vi "41 rec.vi"() -> ()   [LabVIEW 2014]
uses:
  <vilib>/LabVIEW Targets/FPGA/cRIO/shared/nicrio_ModuleControls/nicrio_cRIO-9467_Altitude.ctl
  <vilib>/LabVIEW Targets/FPGA/cRIO/shared/nicrio_ModuleControls/nicrio_cRIO-9467_Longitude.ctl
  <vilib>/LabVIEW Targets/FPGA/cRIO/shared/nicrio_ModuleControls/nicrio_cRIO-9467_Latitude.ctl
  <vilib>/LabVIEW Targets/FPGA/cRIO/shared/nicrio_ModuleControls/nicrio_cRIO-9225_DataRatesRing.ctl
  <vilib>/LabVIEW Targets/FPGA/cRIO/shared/nicrio_ModuleControls/nicrio_cRIO-9227_DataRatesRing.ctl
  <vilib>/rvi/FXPMathLib/FxpSinAndCos/subVIs/nifxpmath_SinAndCos_SimConfig.ctl
  <vilib>/rvi/FXPMathLib/FxpRectToPolar/subVIs/nifxpmath_RectToPolar_SimConfig.ctl
  <vilib>/rvi/Emulation/niFpgaGetClockAttributes.vi
  <vilib>/rvi/Emulation/niFpgaSctlEmulationGetInTimedLoop.vi
  <vilib>/rvi/Emulation/niFpgaEmulationReportErrorSimple.vi
  <vilib>/rvi/eio/common/nirviEmuTemplateMethod_errors.vi
  <vilib>/rvi/eio/common/nirviEmuTemplatePropertyGet_noerrors.vi
  <vilib>/rvi/Emulation/niFpgaCriticalErrorInLSC.vi
  <vilib>/rvi/Memory/Memory_Emulation/nirvimemoryFastEmulation.vi
  <vilib>/rvi/Memory/Memory_Emulation/nirvimemoryEmulation.vi
  <vilib>/rvi/Emulation/niFpgaEmulationIsFPGAContextNoSignature.vi
  <vilib>/rvi/DataTransferAndStorage/Container/Common/niFpgaContainerGetUniqueNameForEmu.vi
  <vilib>/rvi/Emulation/niFpgaProcessEmulError.vi
  <vilib>/rvi/errors/nirviReportUnexpectedCaseInternalError (U32).vi
  <vilib>/rvi/FXPMathLib/FxpSinAndCos/simVIs/DllFxpSinAndCosTemp_sub.vi
  <vilib>/rvi/FXPMathLib/FxpRectToPolar/simVIs/DllFxpRectToPolarTemp_sub.vi
  <vilib>/rvi/eio/common/nirviEmuTemplatePropertyGet_errors.vi
  <vilib>/rvi/DataTransferAndStorage/Container/Common/niFpgaContainerSetEmuInfo.vi
  <vilib>/rvi/eio/common/nirviEmuReportErrorAndStop.vi
  <vilib>/rvi/eio/common/nirviEmuTemplatePropertySet_noerrors.vi
  <vilib>/eio/EIOMethodNode/EIOMethodNode.xnode
  <vilib>/eio/EIOPropertyNode/EIOPropertyNode.xnode
  <vilib>/eio/EIONode/EIONode.xnode
  <vilib>/rvi/DataTransferAndStorage/Container/XNode/niFpgaContainer.xnode
  <vilib>/rvi/FXPMathLib/FxpMul/XNode/nifxpmath_Multiplier.xnode
  <vilib>/rvi/FXPMathLib/FxpSinAndCos/XNode/nifxpmath_SinAndCos.xnode
  <vilib>/rvi/FXPMathLib/FxpAdd/XNode/nifxpmath_Add.xnode
  <vilib>/rvi/FXPMathLib/FxpSub/XNode/nifxpmath_Sub.xnode
  <vilib>/rvi/FXPMathLib/FxpRectToPolar/XNode/nifxpmath_RectToPolar.xnode
  <vilib>/rvi/LocalResourceManager/LocalResourceManager.xnode
  <vilib>/rvi/FXPMathLib/sim/FxpSim.dll
  akhil/fpga timekeeper/FPGA Timekeeper.lvlib
  <vilib>/rvi/eio/common/nirviEmuTemplatePropertySet_errors.vi
panel:
  out "angles":fxp<+/-,22,10>[](array[numeric])
  out "Array":T1(array[cluster])
  out "magnitude":fxp<+,60,17>[](array[numeric])
  out "Firmware Version":u32 format="%.0x"
  out "Vendor ID":u16 format="%.0x"
  out "Module ID":u16 format="%.0x"
  out "Serial Number":u32 format="%.0x"
  out "FPGA Error Out":errorcluster
  in  "stop 2":bool
  out "PPS Timestamp (TAI)":u64
  out "UTC Offset":i8
  out "UTC Offset Valid":bool
  out "GPS Status":T2(ring)
  out "Antenna Status":T3(ring)
  out "Leap Second Direction":enum8{"Add", "Delete"}(ring)
  out "Leap Second Pending":bool
  out "Leap Second Occurred":bool
  out "Satellites Available":u8
  out "Self-Survey Complete":bool
  out "Latitude (°)":T4 format="%.6f"
  out "Longitude (°)":T5 format="%.6g"
  out "Altitude (m)":T6 format="%.2f"
  out "Timed Out":bool
  out "Iterations":i32
  out "FPGA Timekeeper time (ns) 2":u64
  out "GPS status":T2(ring)
  out "FPGA Timekeeper locked":bool
  out "offset from time reference":i32
  out "antenna status":T3(ring)
  out "satellites available":u8
  out "UTC offset":i8
  out "UTC offset valid":bool
  out "ROCOF voltage":fxp<+/-,26,12>
  out "ROCOF current":fxp<+/-,26,12>
  out "DIFFERENCE IN ANGLES":fxp<+/-,26,12>
  out "DIFFERENCE IN ANGLES 2":fxp<+/-,26,12>
  out "Voltage Frequency":fxp<+/-,49,18>
  out "Current Frequency":fxp<+/-,49,18>
  in  "stop":bool
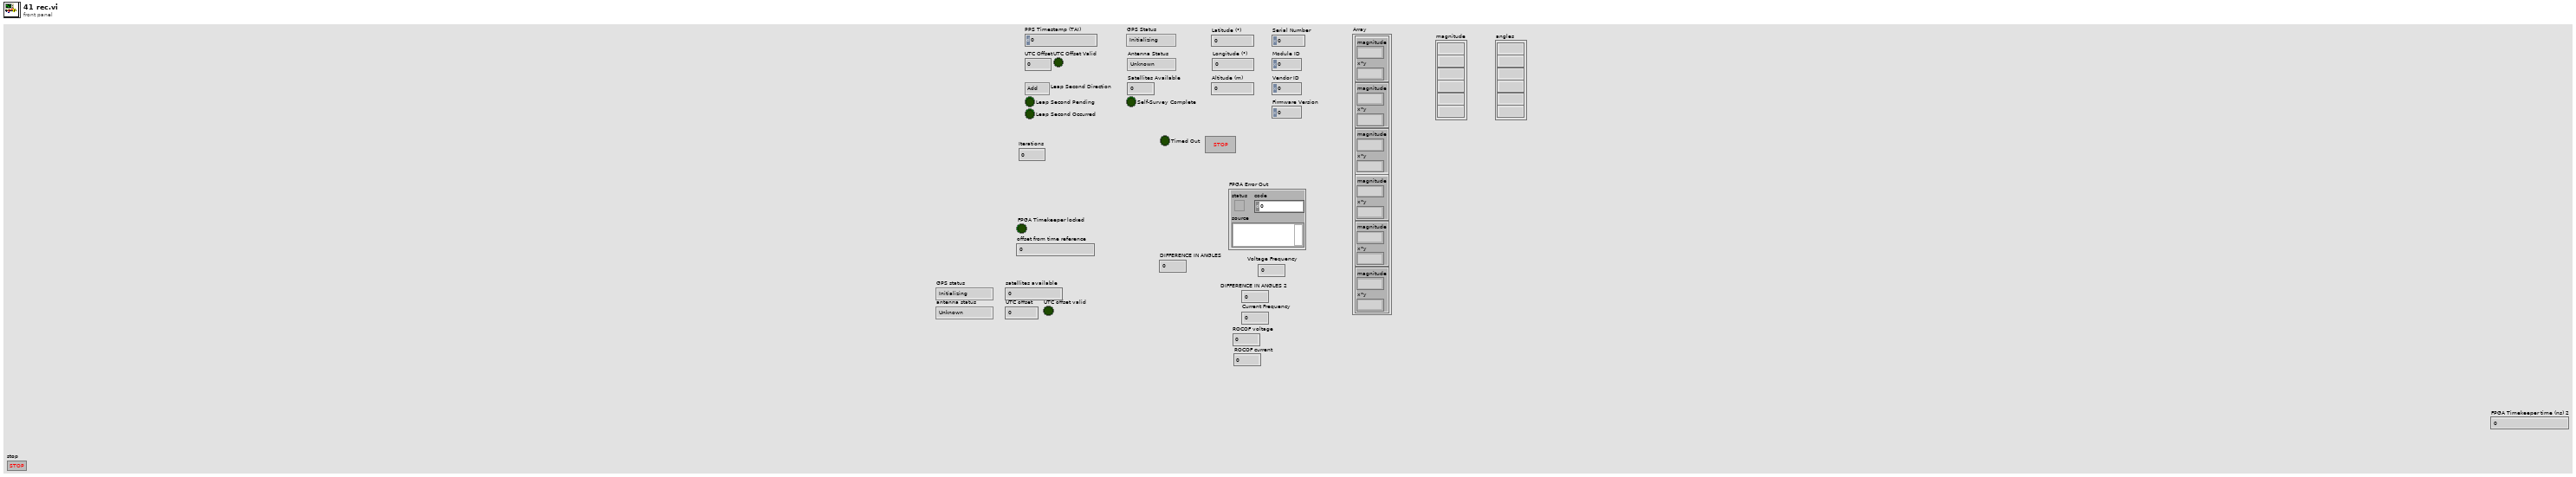
[diagram p1: front panel]
types:
  T1 = cluster{"magnitude":fxp<+,60,17>, "x*y":fxp<+/-,22,10>}[]
  T2 = enum8{"Initializing", "Normal", "Unable to get fix"}
  T3 = enum8{"Unknown", "Normal", "Absent", "Overcurrent"}
  T4 = typedef "nicrio_cRIO-9467_Latitude.ctl" = fxp<+/-,28,8>
  T5 = typedef "nicrio_cRIO-9467_Longitude.ctl" = fxp<+/-,29,9>
  T6 = typedef "nicrio_cRIO-9467_Altitude.ctl" = fxp<+/-,24,17>
  T7 = typedef "nicrio_cRIO-9227_DataRatesRing.ctl" = u8
  T8 = typedef "nicrio_cRIO-9225_DataRatesRing.ctl" = u8
  T9 = cluster{"magnitude":fxp<+,60,17>, "x*y":fxp<+/-,22,10>}
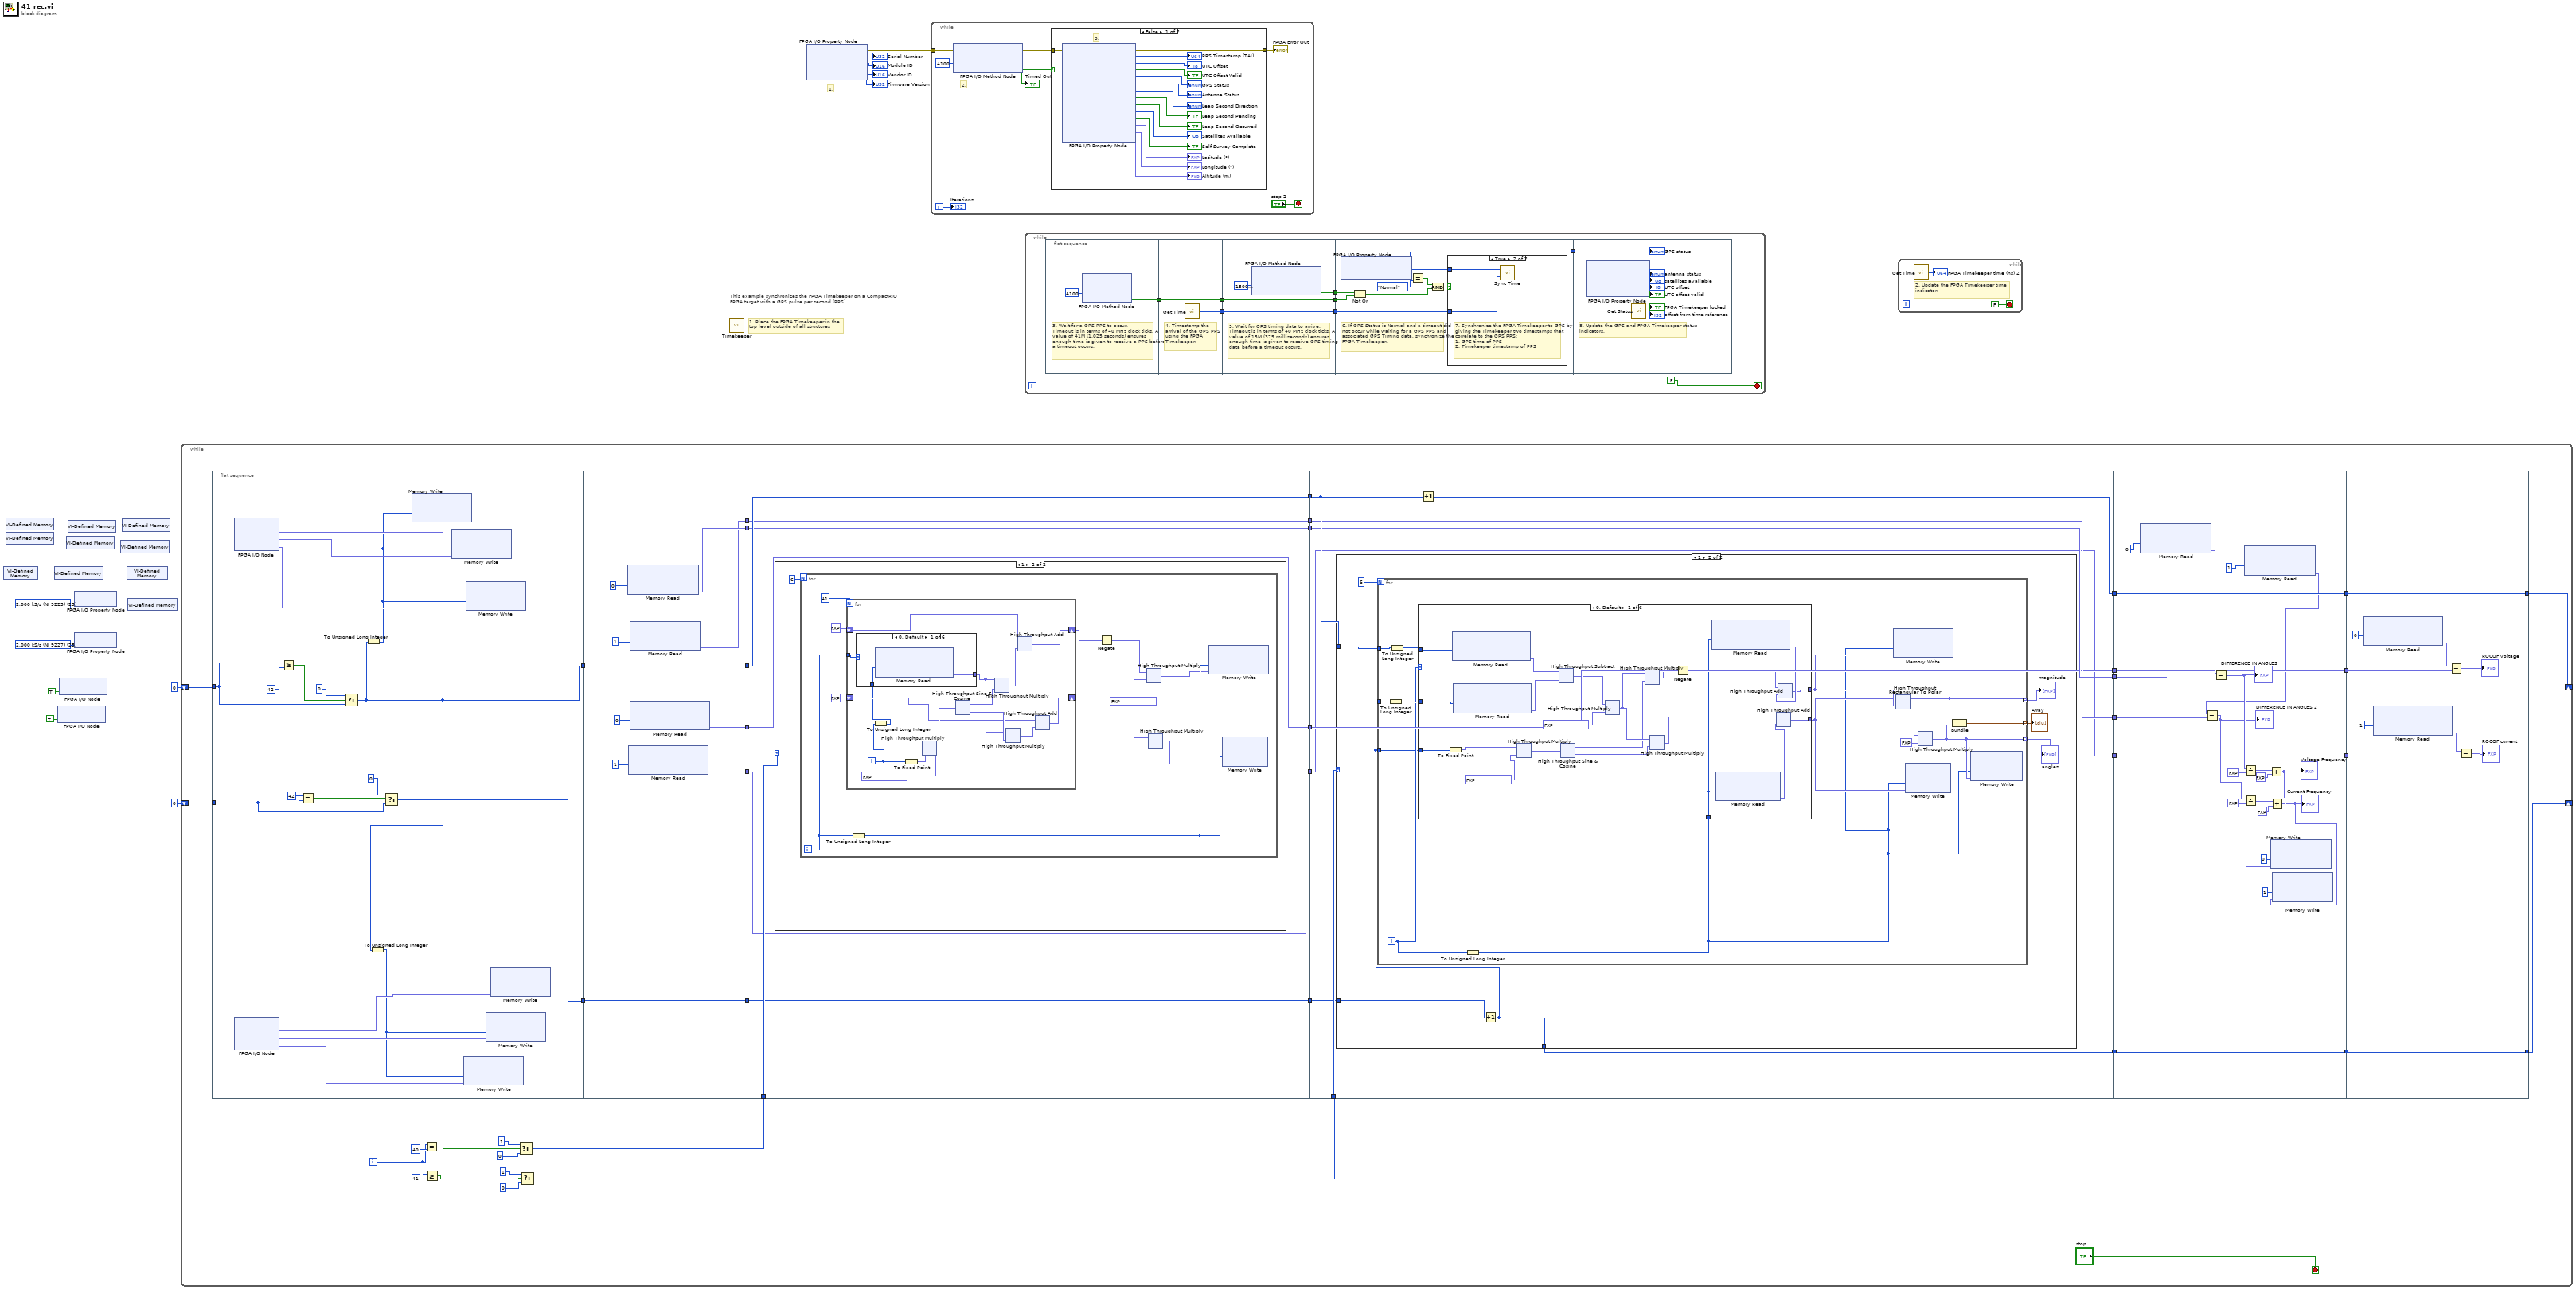
[diagram p0: block diagram]
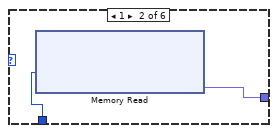
[diagram p5: hidden frame]
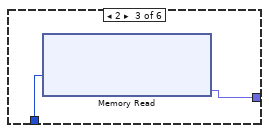
[diagram p6: hidden frame]
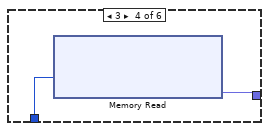
[diagram p7: hidden frame]
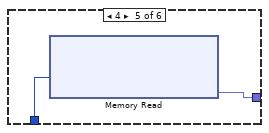
[diagram p8: hidden frame]
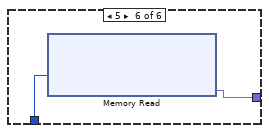
[diagram p9: hidden frame]
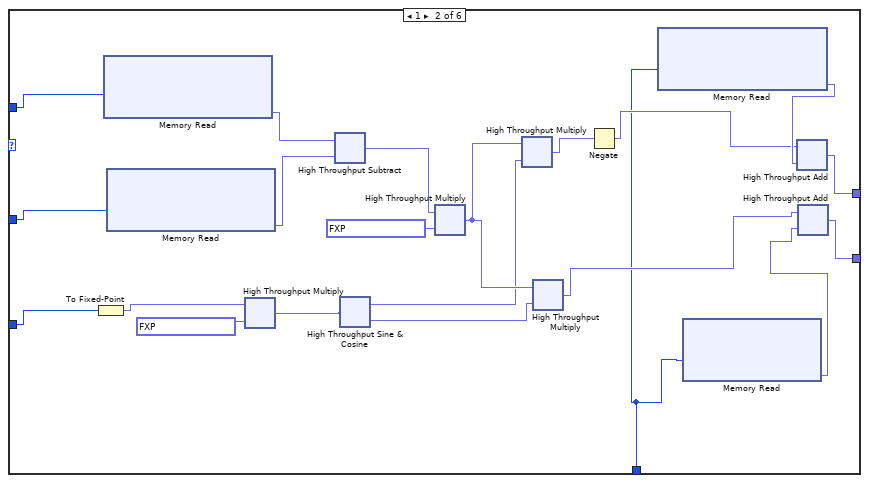
[diagram p11: hidden frame]
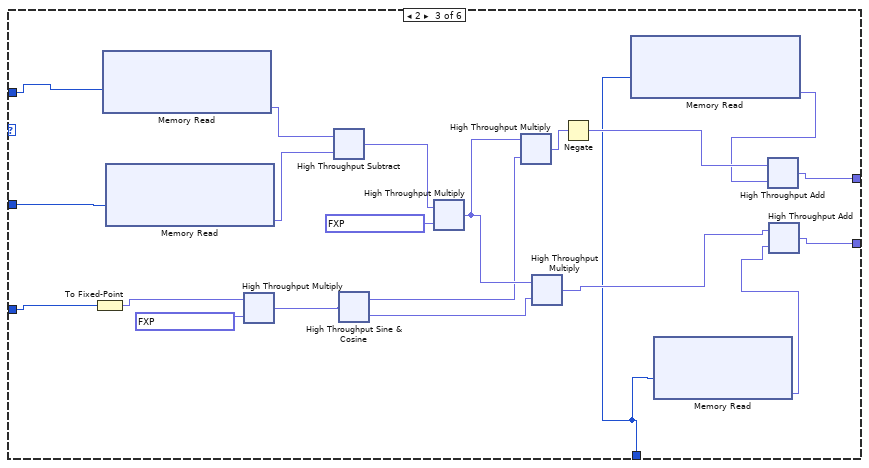
[diagram p12: hidden frame]
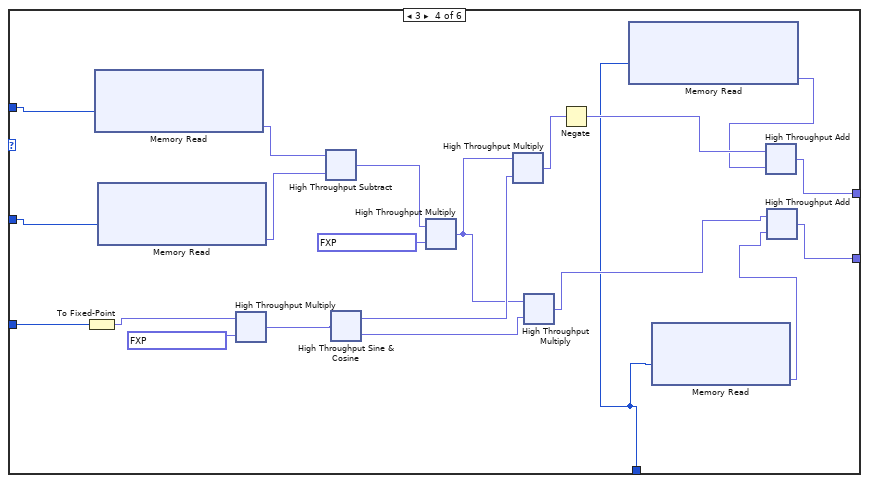
[diagram p13: hidden frame]
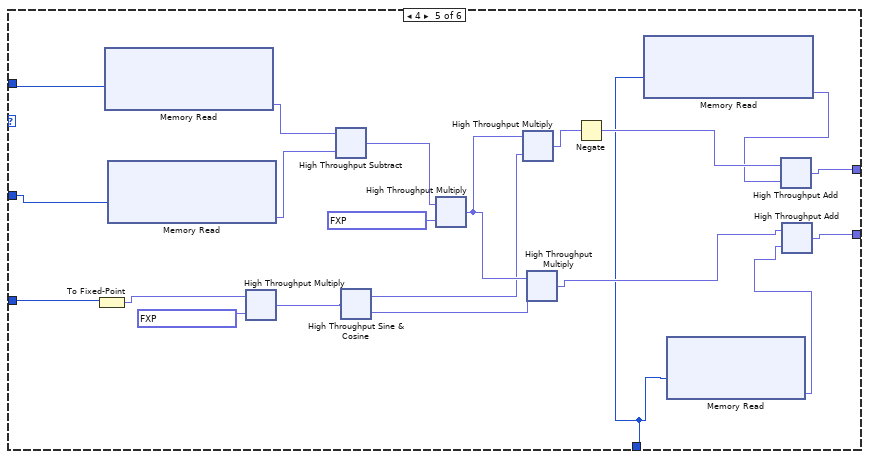
[diagram p14: hidden frame]
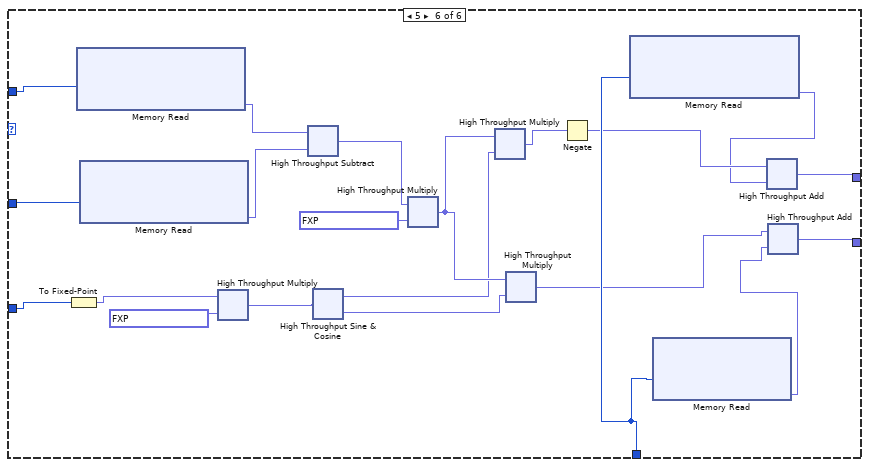
[diagram p15: hidden frame]
diagram:
  w5 = T7 25 items=["50.000 kS/s (NI 9227)"=1, "25.000 kS/s (NI 9227)"=2, "16.667 kS/s (NI 9227)"=3, "12.500 kS/s (NI 9227)"=4, "10.000 kS/s (NI 9227)"=5, "8.333 kS/s (NI 9227)"=6, "7.143 kS/s (NI 9227)"=7, "6.250 kS/s (NI 9227)"=8, "5.556 kS/s (NI 9227)"=9, "5.000 kS/s (NI 9227)"=10, "4.545 kS/s (NI 9227)"=11, "4.167 kS/s (NI 9227)"=12, "3.846 kS/s (NI 9227)"=13, "3.571 kS/s (NI 9227)"=14, "3.333 kS/s (NI 9227)"=15, "3.125 kS/s (NI 9227)"=16, "2.941 kS/s (NI 9227)"=17, "2.778 kS/s (NI 9227)"=18, "2.632 kS/s (NI 9227)"=19, "2.500 kS/s (NI 9227)"=20, "2.381 kS/s (NI 9227)"=21, "2.273 kS/s (NI 9227)"=22, "2.174 kS/s (NI 9227)"=23, "2.083 kS/s (NI 9227)"=24, "2.000 kS/s (NI 9227)"=25, "1.923 kS/s (NI 9227)"=26, "1.852 kS/s (NI 9227)"=27, "1.786 kS/s (NI 9227)"=28, "1.724 kS/s (NI 9227)"=29, "1.667 kS/s (NI 9227)"=30, "1.613 kS/s (NI 9227)"=31] ("Data Rate")
  w6 = T8 25 items=["50.000 kS/s (NI 9225)"=1, "25.000 kS/s (NI 9225)"=2, "16.667 kS/s (NI 9225)"=3, "12.500 kS/s (NI 9225)"=4, "10.000 kS/s (NI 9225)"=5, "8.333 kS/s (NI 9225)"=6, "7.143 kS/s (NI 9225)"=7, "6.250 kS/s (NI 9225)"=8, "5.556 kS/s (NI 9225)"=9, "5.000 kS/s (NI 9225)"=10, "4.545 kS/s (NI 9225)"=11, "4.167 kS/s (NI 9225)"=12, "3.846 kS/s (NI 9225)"=13, "3.571 kS/s (NI 9225)"=14, "3.333 kS/s (NI 9225)"=15, "3.125 kS/s (NI 9225)"=16, "2.941 kS/s (NI 9225)"=17, "2.778 kS/s (NI 9225)"=18, "2.632 kS/s (NI 9225)"=19, "2.500 kS/s (NI 9225)"=20, "2.381 kS/s (NI 9225)"=21, "2.273 kS/s (NI 9225)"=22, "2.174 kS/s (NI 9225)"=23, "2.083 kS/s (NI 9225)"=24, "2.000 kS/s (NI 9225)"=25, "1.923 kS/s (NI 9225)"=26, "1.852 kS/s (NI 9225)"=27, "1.786 kS/s (NI 9225)"=28, "1.724 kS/s (NI 9225)"=29, "1.667 kS/s (NI 9225)"=30, "1.613 kS/s (NI 9225)"=31] ("Data Rate")
  # "1."
  # "This example synchronizes the FPGA Timekeeper on a CompactRIO FPGA target with a GPS pulse per second (PPS)."
  # "1. Place the FPGA Timekeeper in the\ntop level outside of all structures"
  n1 = xnode "VI-Defined Memory"() -> ()  [unwired: 1 out]
  n2 = xnode "VI-Defined Memory"() -> ()  [unwired: 1 out]
  n3 = xnode "VI-Defined Memory"() -> ()  [unwired: 1 out]
  n4 = xnode "VI-Defined Memory"() -> ()  [unwired: 1 out]
  n5 = xnode "FPGA I/O Node"("Mod2/Start"=TRUE) -> ()  [unwired: 1 in, 1 out]
  n6 = xnode "FPGA I/O Node"("Mod1/Start"=TRUE) -> ()  [unwired: 1 in, 1 out]
  n7 = xnode "VI-Defined Memory"() -> ()  [unwired: 1 out]
  n8 = xnode "VI-Defined Memory"() -> ()  [unwired: 1 out]
  n9 = xnode "FPGA I/O Property Node"("Data Rate"=w6) -> ()  [unwired: 1 in, 1 out]
  n10 = xnode "FPGA I/O Property Node"("Data Rate"=w5) -> ()  [unwired: 1 in, 1 out]
  n11 = xnode "VI-Defined Memory"() -> ()  [unwired: 1 out]
  n12 = xnode "VI-Defined Memory"() -> ()  [unwired: 1 out]
  n13 = xnode "VI-Defined Memory"() -> ()  [unwired: 1 out]
  n14 = xnode "VI-Defined Memory"() -> ()  [unwired: 1 out]
  n15 = while {
    shift-right: [w50] -> _
    shift-left: 0 -> [w51]
    shift-right: [w34] -> _
    shift-left: 0 ("t") -> [w36]
    i -> [w41]
    stop <- "stop" stop-if-true
    n16 = flat-sequence {
      tunnel: w51 -> [w58]
      tunnel: [w52] -> w31
      tunnel: w36 -> [w54]
      tunnel: [w53] -> w29
      tunnel: w31 -> [w79]
      tunnel: [w79] -> w30
      tunnel: w29 -> [w78]
      tunnel: [w78] -> w28
      tunnel: [w75] -> w25
      tunnel: [w74] -> w22
      tunnel: [w71] -> w16
      tunnel: [w70] -> w12
      tunnel: w30 -> [w86]
      tunnel: w40 -> [w85]
      tunnel: [w86] -> w39
      tunnel: [w84] -> w35
      tunnel: w28 -> [w84]
      tunnel: [w83] -> w26
      tunnel: w25 -> [w83]
      tunnel: [w82] -> w23
      tunnel: w22 -> [w82]
      tunnel: [w81] -> w17
      tunnel: w16 -> [w81]
      tunnel: [w80] -> w13
      tunnel: w12 -> [w80]
      tunnel: w39 -> [w162]
      tunnel: w38 -> [w164]
      tunnel: w35 -> [w161]
      tunnel: [w163] -> w33
      tunnel: [w160] -> w32
      tunnel: [w159] -> w27
      tunnel: w26 -> [w159]
      tunnel: [w158] -> w24
      tunnel: w23 -> [w158]
      tunnel: [w157] -> w18
      tunnel: w17 -> [w157]
      tunnel: [w156] -> w14
      tunnel: w13 -> [w156]
      tunnel: w33 -> [w551]
      tunnel: w32 -> [w550]
      tunnel: w27 -> [w540]
      tunnel: w24 -> [w530]
      tunnel: [w551] -> w21
      tunnel: [w550] -> w20
      tunnel: [w533] -> w19
      tunnel: w18 -> [w533]
      tunnel: [w532] -> w15
      tunnel: w14 -> [w532]
      tunnel: [w560] -> w34
      tunnel: [w561] -> w50
      tunnel: w21 -> [w561]
      tunnel: w20 -> [w560]
      tunnel: w19 -> [w555]
      tunnel: w15 -> [w554]
      frame #0 {
        n17 = xnode "FPGA I/O Node"() -> ("Mod1/AI0"=w66:fxp<+/-,24,10>, "Mod1/AI1"=w62:fxp<+/-,24,10>, "Mod1/AI2"=w65:fxp<+/-,24,10>)  [unwired: 3 in, 3 out]
        n18 = xnode "FPGA I/O Node"() -> ("Mod2/AI0"=w69:fxp<+/-,24,5>, "Mod2/AI1"=w68:fxp<+/-,24,5>, "Mod2/AI2"=w67:fxp<+/-,24,5>)  [unwired: 3 in, 3 out]
        n19 = Greater Or Equal?(x=w58, y=42 ("x")) -> (x >= y?=w64:bool)
        n20 = Equal?(x=42, y=w54) -> (x = y?=w56:bool)
        n21 = Select(t=0, s=w64, f=w58) -> (s? t:f=w52:i32)
        n22 = To Unsigned Long Integer(number=w52) -> (unsigned 32bit integer=w61:u32)
        n23 = To Unsigned Long Integer(number=w52) -> (unsigned 32bit integer=w60:u32)
        n24 = Select(t=0, s=w56, f=w54) -> (s? t:f=w53:i32)
        n25 = xnode ("Memory Write")("Address"=w61, "Data"=w66) -> ()  [unwired: 1 in, 1 out]
        n26 = xnode ("Memory Write")("Address"=w61, "Data"=w62) -> ()  [unwired: 1 in, 1 out]
        n27 = xnode ("Memory Write")("Address"=w60, "Data"=w67) -> ()  [unwired: 1 in, 1 out]
        n28 = xnode ("Memory Write")("Address"=w61, "Data"=w65) -> ()  [unwired: 1 in, 1 out]
        n29 = xnode ("Memory Write")("Address"=w60, "Data"=w68) -> ()  [unwired: 1 in, 1 out]
        n30 = xnode ("Memory Write")("Address"=w60, "Data"=w69) -> ()  [unwired: 1 in, 1 out]
      }
      frame #1 {
        n31 = xnode ("Memory Read")("Address"=u32 0) -> ("Data"=w75:fxp<+/-,25,11>)  [unwired: 1 in, 1 out]
        n32 = xnode ("Memory Read")("Address"=u32 1) -> ("Data"=w70:fxp<+/-,25,11>)  [unwired: 1 in, 1 out]
        n33 = xnode ("Memory Read")("Address"=u32 1) -> ("Data"=w74:fxp<+/-,25,11>)  [unwired: 1 in, 1 out]
        n34 = xnode ("Memory Read")("Address"=u32 0) -> ("Data"=w71:fxp<+/-,25,11>)  [unwired: 1 in, 1 out]
      }
      frame #2 {
        n35 = case shown="1" w85 {
          frame 0, Default {
          }
          frame 1 {
            n36 = for {
              N: 6 -> [_]
              i -> [w94]
              w88 = fxp<+/-,16,1> 0.03533935546875 ("y")
              n37 = for {
                N: 41 -> [_]
                shift-right: [w106] -> w92
                shift-left: fxp<+/-,44,16> 0.0 ("x+y") -> [w105]
                shift-right: [w109] -> w95
                shift-left: fxp<+/-,42,14> 0.0 ("x+y") -> [w104]
                tunnel: w94 -> [w103]
                i -> [w101]
                n38 = To Unsigned Long Integer(number=w101) -> (unsigned 32bit integer=w100:u32)
                n39 = case shown="0, Default" w103 {
                  tunnel: [w115 w116 w118 w120 w122 w125] -> w102
                  tunnel: w100 -> [w114 w117 w119 w121 w123 w124]
                  frame 0, Default {
                    n40 = xnode ("Memory Read")("Address"=w114) -> ("Data"=w115:fxp<+/-,25,11>)  [unwired: 1 in, 1 out]
                  }
                  frame 1 {
                    n41 = xnode ("Memory Read")("Address"=w117) -> ("Data"=w116:fxp<+/-,25,11>)  [unwired: 1 in, 1 out]
                  }
                  frame 2 {
                    n42 = xnode ("Memory Read")("Address"=w119) -> ("Data"=w118:fxp<+/-,25,11>)  [unwired: 1 in, 1 out]
                  }
                  frame 3 {
                    n43 = xnode ("Memory Read")("Address"=w121) -> ("Data"=w120:fxp<+/-,25,11>)  [unwired: 1 in, 1 out]
                  }
                  frame 4 {
                    n44 = xnode ("Memory Read")("Address"=w123) -> ("Data"=w122:fxp<+/-,25,11>)  [unwired: 1 in, 1 out]
                  }
                  frame 5 {
                    n45 = xnode ("Memory Read")("Address"=w124) -> ("Data"=w125:fxp<+/-,25,11>)  [unwired: 1 in, 1 out]
                  }
                }
                n46 = To Fixed-Point(number=w101) -> (fixed-point=w113:fxp<+/-,32,32>)  [unwired: 1 in]
                n47 = xnode ("High Throughput Multiply")("x"=fxp<+/-,32,16> 0.04998779296875 ("number"), "y"=w113) -> ("x*y"=w112:fxp<+/-,64,48>)
                n48 = xnode "High Throughput Sine & Cosine"("x (pi)"=w112) -> ("sin(x)"=w111:fxp<+/-,16,2>, "cos(x)"=w108:fxp<+/-,16,2>)
                n49 = xnode ("High Throughput Multiply")("x"=w102, "y"=w111) -> ("x*y"=w110:fxp<+/-,41,13>)
                n50 = xnode ("High Throughput Multiply")("x"=w102, "y"=w108) -> ("x*y"=w107:fxp<+/-,41,13>)
                n51 = xnode ("High Throughput Add")("x"=w104, "y"=w110) -> ("x+y"=w109:fxp<+/-,42,14>)
                n52 = xnode ("High Throughput Add")("x"=w105, "y"=w107) -> ("x+y"=w106:fxp<+/-,44,16>)
              }
              n53 = To Unsigned Long Integer(number=w94) -> (unsigned 32bit integer=w93:u32)
              n54 = Negate(x=w95) -> (-x=w91:fxp<+/-,43,15>)
              n55 = xnode ("High Throughput Multiply")("x"=w91, "y"=w88) -> ("x*y"=w89:fxp<+/-,59,16>)
              n56 = xnode ("High Throughput Multiply")("x"=w88, "y"=w92) -> ("x*y"=w90:fxp<+/-,60,17>)
              n57 = xnode ("Memory Write")("Address"=w93, "Data"=w89) -> ()  [unwired: 1 in, 1 out]
              n58 = xnode ("Memory Write")("Address"=w93, "Data"=w90) -> ()  [unwired: 1 in, 1 out]
            }
          }
        }
      }
      frame #3 {
        n59 = case shown="1" w164 {
          tunnel: w162 -> [_ w171]
          tunnel: w161 -> [w165 w167]
          tunnel: [w165 w166] -> w160
          frame 0, Default {
          }
          frame 1 {
            n60 = Increment(x=w167) -> (x+1=w166:i32)
            n61 = for {
              N: 6 -> [_]
              tunnel: w171 -> [w186]
              tunnel: [w178] -> w170 mode=indexing
              tunnel: [w174] -> w168 mode=indexing
              tunnel: [w177] -> w169 mode=indexing
              tunnel: w166 -> [w176]
              tunnel: w166 -> [w175]
              i -> [w183]
              n62 = To Unsigned Long Integer(number=w176) -> (unsigned 32bit integer=w184:u32)
              n63 = To Unsigned Long Integer(number=w186) -> (unsigned 32bit integer=w185:u32)
              n64 = To Unsigned Long Integer(number=w183) -> (unsigned 32bit integer=w173:u32)
              n65 = case shown="0, Default" w183 {
                tunnel: w185 -> [w244 w284 w335 w386 w438 w488]
                tunnel: w184 -> [w243 w283 w336 w387 w437 w487]
                tunnel: w173 -> [w230 w278 w329 w380 w431 w486]
                tunnel: [w228 w277 w328 w379 w430 w481] -> w180
                tunnel: [w227 w276 w327 w378 w429 w480] -> w179
                tunnel: w175 -> [w226 w275 w326 w377 w428 w479]
                frame 0, Default {
                  n66 = To Fixed-Point(number=w226) -> (fixed-point=w237:fxp<+/-,32,32>)  [unwired: 1 in]
                  n67 = xnode ("Memory Read")("Address"=w244) -> ("Data"=w235:fxp<+/-,25,11>)  [unwired: 1 in, 1 out]
                  n68 = xnode ("Memory Read")("Address"=w243) -> ("Data"=w234:fxp<+/-,25,11>)  [unwired: 1 in, 1 out]
                  n69 = xnode ("High Throughput Multiply")("x"=w237, "y"=fxp<+/-,32,16> 0.04998779296875 ("number")) -> ("x*y"=w236:fxp<+/-,64,48>)
                  n70 = xnode "High Throughput Subtract"("x"=w235, "y"=w234) -> ("x-y"=w242:fxp<+/-,26,12>)
                  n71 = xnode "High Throughput Sine & Cosine"("x (pi)"=w236) -> ("sin(x)"=w239:fxp<+/-,16,2>, "cos(x)"=w238:fxp<+/-,16,2>)
                  n72 = xnode ("High Throughput Multiply")("x"=w242, "y"=fxp<+/-,16,1> 0.03533935546875) -> ("x*y"=w241:fxp<+/-,42,13>)
                  n73 = xnode ("High Throughput Multiply")("x"=w241, "y"=w239) -> ("x*y"=w240:fxp<+/-,58,15>)
                  n74 = xnode ("High Throughput Multiply")("x"=w241, "y"=w238) -> ("x*y"=w229:fxp<+/-,58,15>)
                  n75 = Negate(x=w240) -> (-x=w231:fxp<+/-,59,16>)
                  n76 = xnode ("Memory Read")("Address"=w230) -> ("Data"=w232:fxp<+/-,25,11>)  [unwired: 1 in, 1 out]
                  n77 = xnode ("Memory Read")("Address"=w230) -> ("Data"=w233:fxp<+/-,25,11>)  [unwired: 1 in, 1 out]
                  n78 = xnode ("High Throughput Add")("x"=w229, "y"=w233) -> ("x+y"=w227:fxp<+/-,59,16>)
                  n79 = xnode ("High Throughput Add")("x"=w231, "y"=w232) -> ("x+y"=w228:fxp<+/-,60,17>)
                }
                frame 1 {
                  n80 = To Fixed-Point(number=w275) -> (fixed-point=w289:fxp<+/-,32,32>)  [unwired: 1 in]
                  n81 = xnode ("Memory Read")("Address"=w284) -> ("Data"=w286:fxp<+/-,25,11>)  [unwired: 1 in, 1 out]
                  n82 = xnode ("Memory Read")("Address"=w283) -> ("Data"=w285:fxp<+/-,25,11>)  [unwired: 1 in, 1 out]
                  n83 = xnode ("High Throughput Multiply")("x"=w289, "y"=fxp<+/-,16,1> 0.04998779296875) -> ("x*y"=w287:fxp<+/-,48,33>)
                  n84 = xnode "High Throughput Subtract"("x"=w286, "y"=w285) -> ("x-y"=w295:fxp<+/-,26,12>)
                  n85 = xnode "High Throughput Sine & Cosine"("x (pi)"=w287) -> ("sin(x)"=w291:fxp<+/-,16,2>, "cos(x)"=w290:fxp<+/-,16,2>)
                  n86 = xnode ("High Throughput Multiply")("x"=w295, "y"=fxp<+/-,16,1> 0.03533935546875) -> ("x*y"=w293:fxp<+/-,42,13>)
                  n87 = xnode ("High Throughput Multiply")("x"=w293, "y"=w291) -> ("x*y"=w292:fxp<+/-,58,15>)
                  n88 = xnode ("High Throughput Multiply")("x"=w293, "y"=w290) -> ("x*y"=w279:fxp<+/-,58,15>)
                  n89 = Negate(x=w292) -> (-x=w280:fxp<+/-,59,16>)
                  n90 = xnode ("Memory Read")("Address"=w278) -> ("Data"=w281:fxp<+/-,25,11>)  [unwired: 1 in, 1 out]
                  n91 = xnode ("Memory Read")("Address"=w278) -> ("Data"=w282:fxp<+/-,25,11>)  [unwired: 1 in, 1 out]
                  n92 = xnode ("High Throughput Add")("x"=w280, "y"=w281) -> ("x+y"=w277:fxp<+/-,60,17>)
                  n93 = xnode ("High Throughput Add")("x"=w279, "y"=w282) -> ("x+y"=w276:fxp<+/-,59,16>)
                }
                frame 2 {
                  n94 = To Fixed-Point(number=w326) -> (fixed-point=w341:fxp<+/-,32,32>)  [unwired: 1 in]
                  n95 = xnode ("Memory Read")("Address"=w335) -> ("Data"=w338:fxp<+/-,25,11>)  [unwired: 1 in, 1 out]
                  n96 = xnode ("Memory Read")("Address"=w336) -> ("Data"=w337:fxp<+/-,25,11>)  [unwired: 1 in, 1 out]
                  n97 = xnode ("High Throughput Multiply")("x"=w341, "y"=fxp<+/-,16,1> 0.04998779296875) -> ("x*y"=w339:fxp<+/-,48,33>)
                  n98 = xnode "High Throughput Subtract"("x"=w338, "y"=w337) -> ("x-y"=w346:fxp<+/-,26,12>)
                  n99 = xnode "High Throughput Sine & Cosine"("x (pi)"=w339) -> ("sin(x)"=w343:fxp<+/-,16,2>, "cos(x)"=w342:fxp<+/-,16,2>)
                  n100 = xnode ("High Throughput Multiply")("x"=w346, "y"=fxp<+/-,16,1> 0.03533935546875) -> ("x*y"=w344:fxp<+/-,42,13>)
                  n101 = xnode ("High Throughput Multiply")("x"=w344, "y"=w343) -> ("x*y"=w331:fxp<+/-,58,15>)
                  n102 = xnode ("High Throughput Multiply")("x"=w344, "y"=w342) -> ("x*y"=w330:fxp<+/-,58,15>)
                  n103 = Negate(x=w331) -> (-x=w334:fxp<+/-,59,16>)
                  n104 = xnode ("Memory Read")("Address"=w329) -> ("Data"=w332:fxp<+/-,25,11>)  [unwired: 1 in, 1 out]
                  n105 = xnode ("Memory Read")("Address"=w329) -> ("Data"=w333:fxp<+/-,25,11>)  [unwired: 1 in, 1 out]
                  n106 = xnode ("High Throughput Add")("x"=w334, "y"=w332) -> ("x+y"=w328:fxp<+/-,60,17>)
                  n107 = xnode ("High Throughput Add")("x"=w330, "y"=w333) -> ("x+y"=w327:fxp<+/-,59,16>)
                }
                frame 3 {
                  n108 = To Fixed-Point(number=w377) -> (fixed-point=w393:fxp<+/-,32,32>)  [unwired: 1 in]
                  n109 = xnode ("Memory Read")("Address"=w386) -> ("Data"=w396:fxp<+/-,25,11>)  [unwired: 1 in, 1 out]
                  n110 = xnode ("Memory Read")("Address"=w387) -> ("Data"=w397:fxp<+/-,25,11>)  [unwired: 1 in, 1 out]
                  n111 = xnode ("High Throughput Multiply")("x"=w393, "y"=fxp<+/-,16,1> 0.04998779296875) -> ("x*y"=w395:fxp<+/-,48,33>)
                  n112 = xnode "High Throughput Subtract"("x"=w396, "y"=w397) -> ("x-y"=w388:fxp<+/-,26,12>)
                  n113 = xnode "High Throughput Sine & Cosine"("x (pi)"=w395) -> ("sin(x)"=w391:fxp<+/-,16,2>, "cos(x)"=w392:fxp<+/-,16,2>)
                  n114 = xnode ("High Throughput Multiply")("x"=w388, "y"=fxp<+/-,16,1> 0.03533935546875) -> ("x*y"=w390:fxp<+/-,42,13>)
                  n115 = xnode ("High Throughput Multiply")("x"=w390, "y"=w391) -> ("x*y"=w382:fxp<+/-,58,15>)
                  n116 = xnode ("High Throughput Multiply")("x"=w390, "y"=w392) -> ("x*y"=w381:fxp<+/-,58,15>)
                  n117 = Negate(x=w382) -> (-x=w385:fxp<+/-,59,16>)
                  n118 = xnode ("Memory Read")("Address"=w380) -> ("Data"=w383:fxp<+/-,25,11>)  [unwired: 1 in, 1 out]
                  n119 = xnode ("Memory Read")("Address"=w380) -> ("Data"=w384:fxp<+/-,25,11>)  [unwired: 1 in, 1 out]
                  n120 = xnode ("High Throughput Add")("x"=w385, "y"=w383) -> ("x+y"=w379:fxp<+/-,60,17>)
                  n121 = xnode ("High Throughput Add")("x"=w381, "y"=w384) -> ("x+y"=w378:fxp<+/-,59,16>)
                }
                frame 4 {
                  n122 = To Fixed-Point(number=w428) -> (fixed-point=w443:fxp<+/-,32,32>)  [unwired: 1 in]
                  n123 = xnode ("Memory Read")("Address"=w438) -> ("Data"=w440:fxp<+/-,25,11>)  [unwired: 1 in, 1 out]
                  n124 = xnode ("Memory Read")("Address"=w437) -> ("Data"=w439:fxp<+/-,25,11>)  [unwired: 1 in, 1 out]
                  n125 = xnode ("High Throughput Multiply")("x"=w443, "y"=fxp<+/-,16,1> 0.04998779296875) -> ("x*y"=w441:fxp<+/-,48,33>)
                  n126 = xnode "High Throughput Subtract"("x"=w440, "y"=w439) -> ("x-y"=w448:fxp<+/-,26,12>)
                  n127 = xnode "High Throughput Sine & Cosine"("x (pi)"=w441) -> ("sin(x)"=w445:fxp<+/-,16,2>, "cos(x)"=w444:fxp<+/-,16,2>)
                  n128 = xnode ("High Throughput Multiply")("x"=w448, "y"=fxp<+/-,16,1> 0.03533935546875) -> ("x*y"=w446:fxp<+/-,42,13>)
                  n129 = xnode ("High Throughput Multiply")("x"=w446, "y"=w445) -> ("x*y"=w433:fxp<+/-,58,15>)
                  n130 = xnode ("High Throughput Multiply")("x"=w446, "y"=w444) -> ("x*y"=w432:fxp<+/-,58,15>)
                  n131 = Negate(x=w433) -> (-x=w436:fxp<+/-,59,16>)
                  n132 = xnode ("Memory Read")("Address"=w431) -> ("Data"=w434:fxp<+/-,25,11>)  [unwired: 1 in, 1 out]
                  n133 = xnode ("Memory Read")("Address"=w431) -> ("Data"=w435:fxp<+/-,25,11>)  [unwired: 1 in, 1 out]
                  n134 = xnode ("High Throughput Add")("x"=w436, "y"=w434) -> ("x+y"=w430:fxp<+/-,60,17>)
                  n135 = xnode ("High Throughput Add")("x"=w432, "y"=w435) -> ("x+y"=w429:fxp<+/-,59,16>)
                }
                frame 5 {
                  n136 = To Fixed-Point(number=w479) -> (fixed-point=w493:fxp<+/-,32,32>)  [unwired: 1 in]
                  n137 = xnode ("Memory Read")("Address"=w488) -> ("Data"=w490:fxp<+/-,25,11>)  [unwired: 1 in, 1 out]
                  n138 = xnode ("Memory Read")("Address"=w487) -> ("Data"=w489:fxp<+/-,25,11>)  [unwired: 1 in, 1 out]
                  n139 = xnode ("High Throughput Multiply")("x"=w493, "y"=fxp<+/-,16,1> 0.04998779296875) -> ("x*y"=w491:fxp<+/-,48,33>)
                  n140 = xnode "High Throughput Subtract"("x"=w490, "y"=w489) -> ("x-y"=w499:fxp<+/-,26,12>)
                  n141 = xnode "High Throughput Sine & Cosine"("x (pi)"=w491) -> ("sin(x)"=w495:fxp<+/-,16,2>, "cos(x)"=w494:fxp<+/-,16,2>)
                  n142 = xnode ("High Throughput Multiply")("x"=w499, "y"=fxp<+/-,16,1> 0.03533935546875) -> ("x*y"=w497:fxp<+/-,42,13>)
                  n143 = xnode ("High Throughput Multiply")("x"=w497, "y"=w495) -> ("x*y"=w496:fxp<+/-,58,15>)
                  n144 = xnode ("High Throughput Multiply")("x"=w497, "y"=w494) -> ("x*y"=w483:fxp<+/-,58,15>)
                  n145 = Negate(x=w496) -> (-x=w485:fxp<+/-,59,16>)
                  n146 = xnode ("Memory Read")("Address"=w486) -> ("Data"=w482:fxp<+/-,25,11>)  [unwired: 1 in, 1 out]
                  n147 = xnode ("Memory Read")("Address"=w486) -> ("Data"=w484:fxp<+/-,25,11>)  [unwired: 1 in, 1 out]
                  n148 = xnode ("High Throughput Add")("x"=w485, "y"=w482) -> ("x+y"=w481:fxp<+/-,60,17>)
                  n149 = xnode ("High Throughput Add")("x"=w483, "y"=w484) -> ("x+y"=w480:fxp<+/-,59,16>)
                }
              }
              n150 = xnode ("Memory Write")("Address"=w173, "Data"=w180) -> ()  [unwired: 1 in, 1 out]
              n151 = xnode "High Throughput Rectangular To Polar"("x"=w179, "y"=w180) -> ("magnitude"=w178:fxp<+,60,17>, "phase (pi)"=w182:fxp<+/-,16,2>)
              n152 = xnode ("Memory Write")("Address"=w173, "Data"=w179) -> ()  [unwired: 1 in, 1 out]
              n153 = xnode ("High Throughput Multiply")("x"=w182, "y"=fxp<+,6,8> 180.0) -> ("x*y"=w174:fxp<+/-,22,10>)
              n154 = Bundle("magnitude"=w178, "x*y"=w174) -> (w177:T9)  [unwired: 1 in]
              n155 = xnode ("Memory Write")("Address"=w173, "Data"=w174) -> ()  [unwired: 1 in, 1 out]
            }
            "magnitude" <- w170
            "Array" <- w169
            "angles" <- w168
          }
        }
        n156 = Increment(x=w162) -> (x+1=w163:i32)
      }
      frame #4 {
        n157 = xnode ("Memory Read")("Address"=u32 0) -> ("Data"=w541:fxp<+/-,25,11>)  [unwired: 1 in, 1 out]
        n158 = Subtract(x=w541, y=w540) -> (x-y=w539:fxp<+/-,26,12>)
        "DIFFERENCE IN ANGLES" <- w539
        n159 = Divide(x=w539, y=fxp<+/-,17,17> 360.0) -> (x/y=w547:fxp<+/-,43,12>)
        n160 = xnode ("Memory Read")("Address"=u32 1) -> ("Data"=w531:fxp<+/-,25,11>)  [unwired: 1 in, 1 out]
        n161 = Subtract(x=w531, y=w530) -> (x-y=w538:fxp<+/-,26,12>)
        "DIFFERENCE IN ANGLES 2" <- w538
        n162 = Divide(x=w538, y=fxp<+/-,17,17> 360.0) -> (x/y=w545:fxp<+/-,43,12>)
        n163 = Add(x=w547, y=fxp<+/-,34,17> 50.0) -> (x+y=w535:fxp<+/-,49,18>)
        "Voltage Frequency" <- w535
        n164 = Add(x=w545, y=fxp<+/-,34,17> 50.0) -> (x+y=w534:fxp<+/-,49,18>)
        "Current Frequency" <- w534
        n165 = xnode ("Memory Write")("Address"=u32 0, "Data"=w535) -> ()  [unwired: 1 in, 1 out]
        n166 = xnode ("Memory Write")("Address"=u32 1, "Data"=w534) -> ()  [unwired: 1 in, 1 out]
      }
      frame #5 {
        n167 = xnode ("Memory Read")("Address"=u32 0) -> ("Data"=w559:fxp<+/-,25,11>)  [unwired: 1 in, 1 out]
        n168 = xnode ("Memory Read")("Address"=u32 1) -> ("Data"=w557:fxp<+/-,25,11>)  [unwired: 1 in, 1 out]
        n169 = Subtract(x=w559, y=w555) -> (x-y=→"ROCOF voltage":fxp<+/-,26,12>)
        n170 = Subtract(x=w557, y=w554) -> (x-y=→"ROCOF current":fxp<+/-,26,12>)
      }
    }
    n171 = Equal?(x=w41, y=40) -> (x = y?=w42:bool)
    n172 = Greater Or Equal?(x=w41, y=41) -> (x >= y?=w49:bool)
    n173 = Select(t=1, s=w42, f=0) -> (s? t:f=w40:i32)
    n174 = Select(t=1, s=w49, f=0) -> (s? t:f=w38:i32)
  }
  n175 = call "Timekeeper.vi"() -> ()  [unwired: 12 in]
  n176 = xnode "FPGA I/O Property Node"() -> ("error out"=w7:errorcluster, "Serial Number"=→"Serial Number":u32, "Module ID"=→"Module ID":u16, "Vendor ID"=→"Vendor ID":u16, "Firmware Version"=→"Firmware Version":u32)  [unwired: 2 in, 1 out]
  n177 = while {
    tunnel: w7 -> [w563]
    i -> [w562]
    stop <- "stop 2" stop-if-true
    # "2."
    n178 = xnode "FPGA I/O Method Node"("error in"=w563, "Timeout"=41000000) -> ("error out"=w568:errorcluster, "Timed Out"=w565:bool)  [unwired: 1 in, 1 out]
    "Timed Out" <- w565
    n179 = case shown="False" w565 {
      tunnel: w568 -> [w583 w584]
      tunnel: [w572 w584] -> w567
      frame False {
        # "3."
        n180 = xnode "FPGA I/O Property Node"("error in"=w583) -> ("error out"=w572:errorcluster, "PPS Timestamp (TAI)"=→"PPS Timestamp (TAI)":u64, "UTC Offset"=→"UTC Offset":i8, "UTC Offset Valid"=→"UTC Offset Valid":bool, "GPS Status"=→"GPS Status":T2, "Antenna Status"=→"Antenna Status":T3, "Leap Second Direction"=→"Leap Second Direction":enum8{"Add", "Delete"}, "Leap Second Pending"=→"Leap Second Pending":bool, "Leap Second Occurred"=→"Leap Second Occurred":bool, "Satellites Available"=→"Satellites Available":u8, "Self-Survey Complete"=→"Self-Survey Complete":bool, "Latitude (°)"=→"Latitude (°)":T4, "Longitude (°)"=→"Longitude (°)":T5, "Altitude (m)"=→"Altitude (m)":T6)  [unwired: 1 in, 1 out]
      }
      frame True {
      }
    }
    "FPGA Error Out" <- w567
    "Iterations" <- w562
  }
  n181 = while {
    stop <- FALSE stop-if-true
    n182 = flat-sequence {
      tunnel: [w593] -> w592
      tunnel: w592 -> [w596]
      tunnel: [w596] -> w591
      tunnel: [w595] -> w590
      tunnel: [w599] -> w589
      tunnel: w591 -> [w598]
      tunnel: [w598] -> w588
      tunnel: w590 -> [w597]
      tunnel: [w597] -> w587
      tunnel: w589 -> [w608]
      tunnel: w588 -> [w607]
      tunnel: w587 -> [w602]
      tunnel: [w601] -> w586
      tunnel: w586 -> [w618]
      frame #0 {
        # "3. Wait for a GPS PPS to occur.\nTimeout is in terms of 40 MHz clock ticks. A value of 41M (1.025 seconds) ensures enough time is given to receive a PPS before a timeout occurs."
        n183 = xnode "FPGA I/O Method Node"("Timeout"=41000000) -> ("Timed Out"=w593:bool)  [unwired: 1 in, 1 out]
      }
      frame #1 {
        # "4. Timestamp the arrival of the GPS PPS using the FPGA Timekeeper."
        n184 = call "Get Time.vi"() -> ("time (ns)"=w595:u64)
      }
      frame #2 {
        # "5. Wait for GPS timing data to arrive.\nTimeout is in terms of 40 MHz clock ticks. A value of 15M (375 milliseconds) ensures enough time is given to receive GPS timing data before a timeout occurs."
        n185 = xnode "FPGA I/O Method Node"("Timeout"=15000000) -> ("Timed Out"=w599:bool)  [unwired: 1 in, 1 out]
      }
      frame #3 {
        # "6. If GPS Status is Normal and a timeout did not occur while waiting for a GPS PPS and associated GPS Timing data, synchronize the FPGA Timekeeper."
        n186 = xnode "FPGA I/O Property Node"() -> ("PPS Timestamp (TAI)"=w603:u64, "GPS Status"=w601:T2)  [unwired: 1 in, 1 out]
        n187 = Not Or(1:w607, 2:w608) -> (0:w605:bool)
        n188 = Equal?(x=w601, y=T2."Normal") -> (x = y?=w606:bool)
        n189 = And(x=w606, y=w605) -> (x .and. y?=w604:bool)
        n190 = case shown="True" w604 {
          tunnel: w603 -> [_ w611]
          tunnel: w602 -> [_ w610]
          frame False {
          }
          frame True {
            # "7. Synchronize the FPGA Timekeeper to GPS by giving the Timekeeper two timestamps that correlate to the GPS PPS:\n1. GPS time of PPS\n2. Timekeeper timestamp of PPS"
            n191 = call "Sync Time.vi"("FPGA Timekeeper time (ns)"=w610, "time reference time (ns)"=w611) -> ()
          }
        }
      }
      frame #4 {
        # "8. Update the GPS and FPGA Timekeeper status indicators."
        n192 = xnode "FPGA I/O Property Node"() -> ("Antenna Status"=→"antenna status":T3, "Satellites Available"=→"satellites available":u8, "UTC Offset"=→"UTC offset":i8, "UTC Offset Valid"=→"UTC offset valid":bool)  [unwired: 1 in, 1 out]
        n193 = call "Get Status.vi"() -> ("FPGA Timekeeper locked"=→"FPGA Timekeeper locked":bool, "offset from time reference"=→"offset from time reference":i32)
        "GPS status" <- w618
      }
    }
  }
  n194 = while {
    stop <- FALSE stop-if-true
    # "2. Update the FPGA Timekeeper time indicator."
    n195 = call "Get Time.vi"() -> ("time (ns)"=→"FPGA Timekeeper time (ns) 2":u64)
  }
